vi "ALTS-2015 Get Cluster to write result in DB.vi"(7 "Options":T2, 8 "error in":errorcluster) -> (0 "error out":errorcluster, 3 "DB Result Cluster Out":T1)   [LabVIEW 2013]
doc: "Copyright © 2005, Soliton Technologies.\nAll rights reserved."
uses:
  Controls/ALTS-2015 write DB Result cases.ctl
  Controls/ALTS-2015 DB Result Cluster.ctl
  Controls/ALTS-2015 Bundle Cluster for DB Result Options.ctl
  Controls/ALTS-2015 LV2GBL WorkOrder&SN Info Options.ctl
panel:
  in  "Simulate DB Result Cluster In":T1={"Sensor_Name"="Sensor 111", "SN"="080925ABR0161", "Work_order_Number"="123", "User1"="U1", "User2"="U2", "User3"="U3", "User4"="U4", "Pressure"=78.79, "Flow"=0.85, "Test_Result"="Pass", "Test_Time"="20100326132520", "Repair Code"=""}
  in  "DB Result Cluster":T1
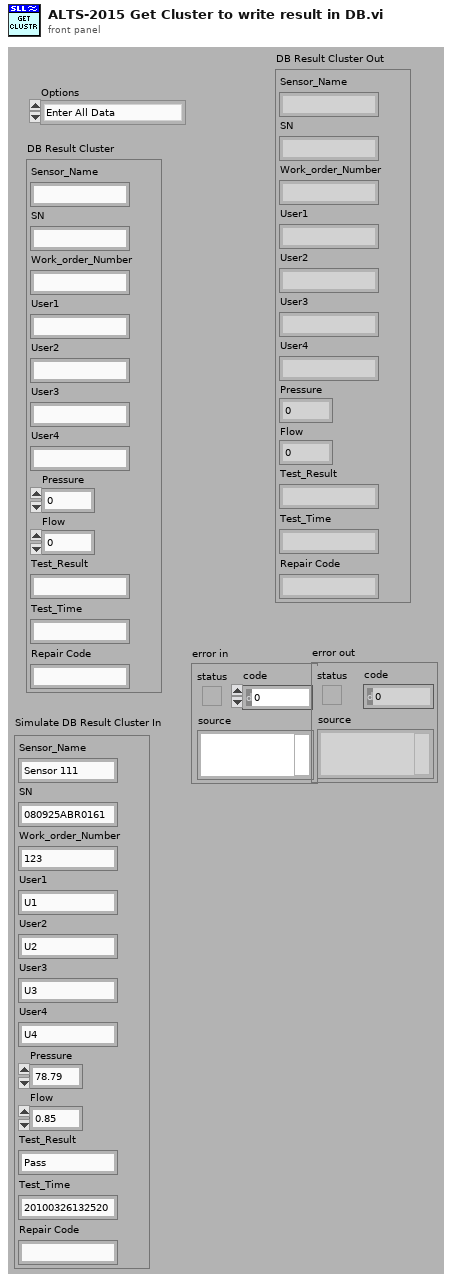
[diagram p1: front panel]
types:
  T1 = typedef "ALTS-2015 DB Result Cluster.ctl" = cluster{"Sensor_Name":string, "SN":string, "Work_order_Number":string, "User1":string, "User2":string, "User3":string, "User4":string, "Pressure":dbl, "Flow":dbl, "Test_Result":string, "Test_Time":string, "Repair Code":string}
  T2 = typedef "ALTS-2015 write DB Result cases.ctl" = enum16{"Enter All Data", "Enter WO & SN"}
  T3 = typedef "ALTS-2015 Bundle Cluster for DB Result Options.ctl" = enum16{"Write", "Read"}
  T4 = typedef "ALTS-2015 LV2GBL WorkOrder&SN Info Options.ctl" = enum16{"Init", "Read all", "Write Work Order", "Write Serial Number", "Clear Serial Number"}
  T5 = typedef "ALTS-2015 WorkOrder&SN Cluster.ctl" = cluster{"Work Order Number":string, "Serial Number":string}
  T6 = typedef "ALTS-2015 User Info Cluster.ctl" = cluster{"User 1":string, "User 2":string, "User 3":string, "User 4":string}
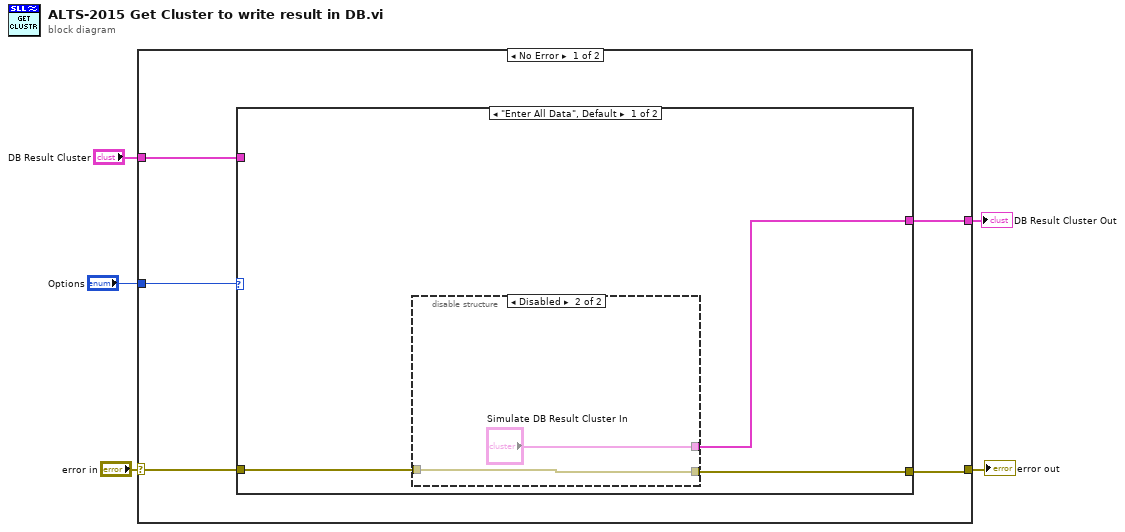
[diagram p0: block diagram]
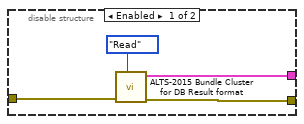
[diagram p2: hidden frame]
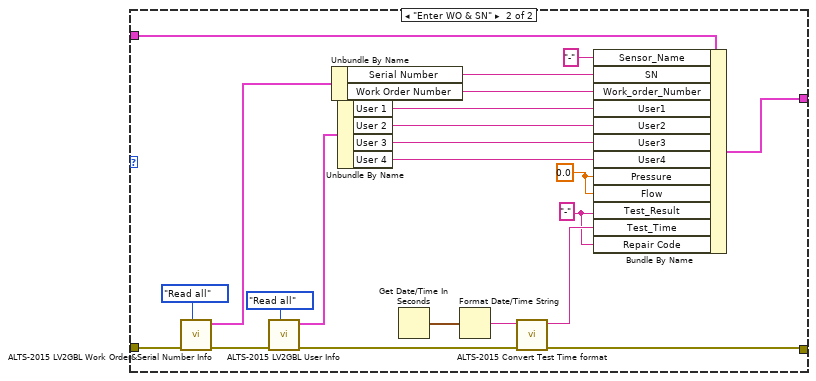
[diagram p3: hidden frame]
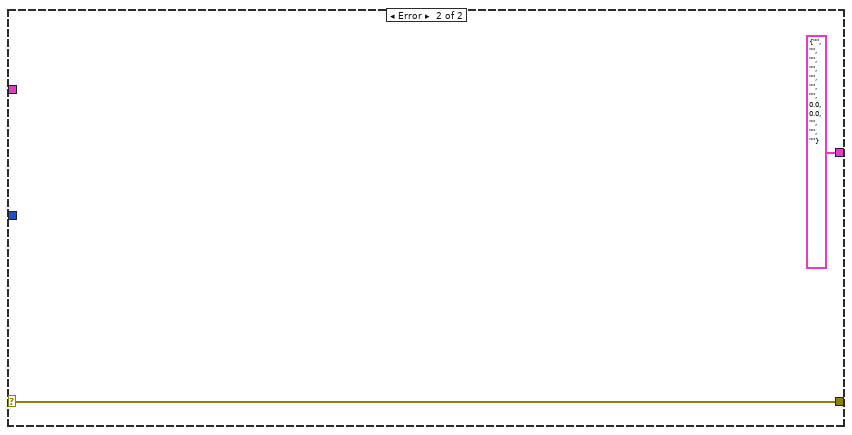
[diagram p4: hidden frame]
diagram:
  n1 = case shown="No Error" "error in" {
    selector: "error in" -> [w9 w43]
    tunnel: [w8 w43] -> w4
    tunnel: "Options" -> [w10 _]
    tunnel: [w7 T1 {"Sensor_Name"="", "SN"="", "Work_order_Number"="", "User1"="", "User2"="", "User3"="", "User4"="", "Pressure"=0.0, "Flow"=0.0, "Test_Result"="", "Test_Time"="", "Repair Code"=""} ("DB Result Cluster Out")] -> w2
    tunnel: "DB Result Cluster" -> [w6 _]
    frame No Error {
      n2 = case shown="\"Enter All Data\", Default" w10 {
        tunnel: w9 -> [w13 w40]
        tunnel: [w12 w36] -> w8
        tunnel: [w11 w41] -> w7
        tunnel: w6 -> [_ w32]
        frame "Enter All Data", Default {
          n3 = disable-structure shown="Disabled" {
            disable-tunnel: w13 -> [w16 w18]
            disable-tunnel: [w15 w18] -> w12
            disable-tunnel: [w14 "Simulate DB Result Cluster In"] -> w11
            frame Enabled {
              n4 = call "ALTS-2015 Bundle Cluster for DB Result format.vi"("Options"=ALTS-2015_Bundle_Cluster_for_DB_Result_Options."Read", "error in (no error)"=w16) -> ("error out"=w15:errorcluster, "DB Result Cluster Out"=w14:T1)  [unwired: 8 in]
            }
            frame Disabled {
            }
          }
        }
        frame "Enter WO & SN" {
          w20 = "-" ("Test_Result")
          w22 = 0.0 ("Pressure")
          n5 = call "ALTS-2015 LV2GBL Work Order&Serial Number Info.vi"("Options"=ALTS-2015_LV2GBL_WorkOrder&SN_Info_Options."Read all", "error in"=w40) -> ("error out"=w24:errorcluster, "Work Order&SN Cluster Out"=w39:T5)  [unwired: 8 in]
          n6 = call "ALTS-2015 LV2GBL User Info.vi"("Options"=enum16{"Read all", "Write all"}."Read all", "error in"=w24) -> ("error out"=w23:errorcluster, "User Info Out"=w31:T6)  [unwired: 8 in]
          n7 = Unbundle By Name(w39) -> ("Serial Number"=w38:string, "Work Order Number"=w37:string)
          n8 = Unbundle By Name(w31) -> ("User 1"=w28:string, "User 2"=w27:string, "User 3"=w26:string, "User 4"=w25:string)
          n9 = Get Date/Time In Seconds() -> (seconds since 1Jan1904=w35:timestamp)
          n10 = Format Date/Time String(seconds (now)=w35) -> (date/time string=w34:string)  [unwired: 2 in]
          n11 = call "ALTS-2015 Convert Test Time format.vi"("error in (no error)"=w23, "String"=w34) -> ("error out"=w36:errorcluster, "Test Time(YYYYMMDDHHMMSS)"=w21:string)  [unwired: 8 in]
          n12 = Bundle By Name(cluster=w32, "Sensor_Name"="-", "SN"=w38, "Work_order_Number"=w37, "User1"=w28, "User2"=w27, "User3"=w26, "User4"=w25, "Pressure"=w22, "Flow"=w22, "Test_Result"=w20, "Test_Time"=w21, "Repair Code"=w20) -> (w41:T1)
        }
      }
    }
    frame Error {
    }
  }
  "error out" <- w4
  "DB Result Cluster Out" <- w2
